vi "WFLastSampleToZeroD.vi"(4 "error in (no error)":errorcluster, 7 "Waveform In":digitalwaveform(waveform)={"t0"=timestamp(0 s since 1904-01-01), "dt"=1.0, "Y"={"transitions"=[], "data"=[]}}) -> (0 "error out":errorcluster, 3 "Waveform Out":digitalwaveform(waveform)={"t0"=timestamp(0 s since 1904-01-01), "dt"=1.0, "Y"={"transitions"=[], "data"=[]}})   [LabVIEW 2013]
uses:
  <vilib>/Waveform/DWDTOps.llb/DWDT Digital Size.vi
  <vilib>/Waveform/DTblOps.llb/DTbl Digital to Boolean Array.vi
  <vilib>/Waveform/DWDTOps.llb/DWDT Boolean Array to Digital.vi
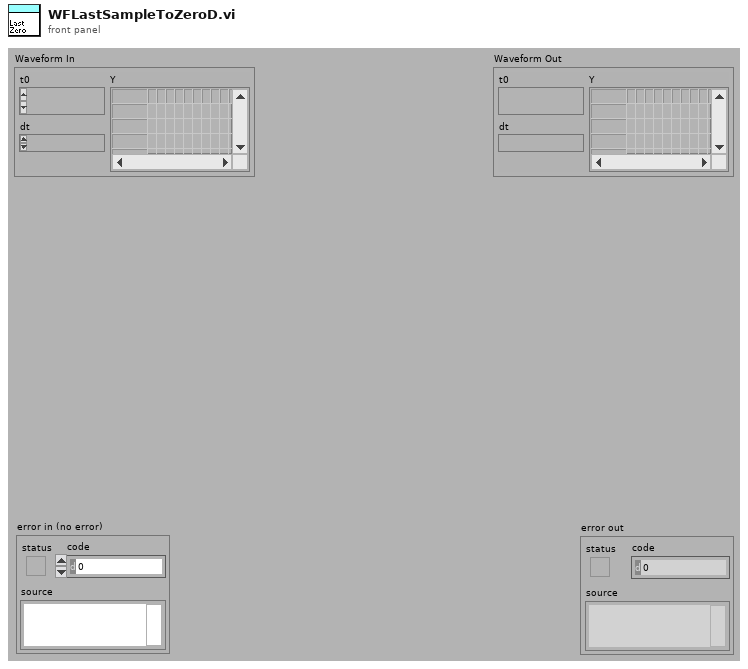
[diagram p1: front panel]
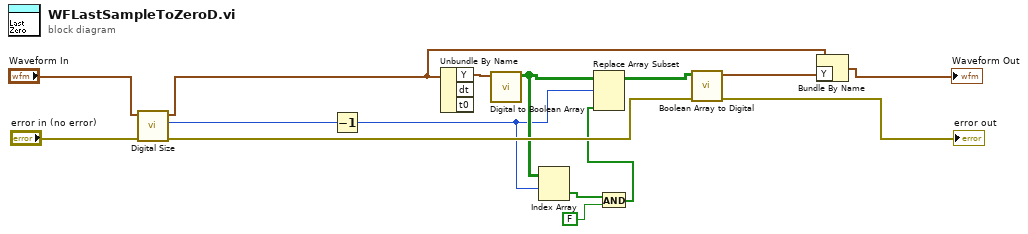
[diagram p0: block diagram]
diagram:
  n1 = call-poly <vilib>:"Digital Size.vi"("error in (no error)"="error in (no error)", "digital waveform in"="Waveform In") -> ("error out"=w6:errorcluster, "number of samples"=w12:i32, "digital waveform out"=w14:digitalwaveform)  [unwired: 6 in, 1 out]
  n2 = Decrement(x=w12) -> (x-1=w4:i32)
  n3 = Unbundle By Name(w14) -> ("Y"=w11:digitaldata)  [unwired: 2 out]
  n4 = call-poly <vilib>:"Digital to Boolean Array.vi"("digital data"=w11) -> ("boolean array"=w5:bool[][])  [unwired: 9 in, 1 out]
  n5 = Index Array(array=w5, index (row)=w4) -> (element=w3:bool[])  [unwired: 1 in]
  n6 = And(x=w3, y=FALSE) -> (x .and. y?=w1:bool[])
  n7 = Replace Array Subset(array=w5, new element=w1, index (row)=w4) -> (w8:bool[][])  [unwired: 1 in]
  n8 = call-poly <vilib>:"Boolean Array to Digital.vi"("error in (no error)"=w6, "boolean array"=w8) -> ("error out"=→"error out":errorcluster, "digital waveform"=w9:digitalwaveform)  [unwired: 8 in]
  n9 = Bundle By Name(cluster=w14, "Y"=w9) -> (→"Waveform Out":digitalwaveform)
